vi "get_output_mode.vi"(8 "error in (no error)":errorcluster, 11 "connection ID":refnum<k5>) -> (0 "error out":errorcluster, 2 "Output mode":T1, 3 "connection ID out":refnum<k5>)   [LabVIEW 2018]
uses:
  typedefs/output_mode.ctl
panel:
  in  "Ouptut modes":string(combo)="0"
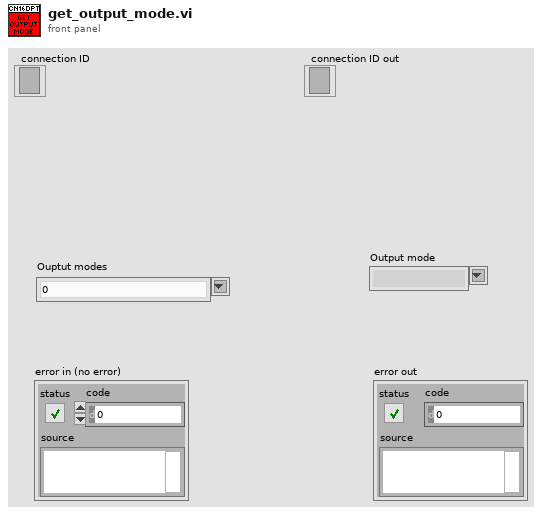
[diagram p1: front panel]
types:
  T1 = typedef "output_mode.ctl" = string
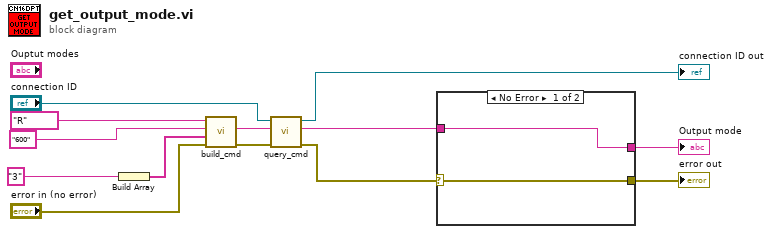
[diagram p0: block diagram]
diagram:
  n1 = Build Array("3" ("Output number")) -> (w2:string[])
  n2 = call "build_cmd.vi"("error in (no error)"="error in (no error)", "Parameter list"=w2, "Command ID"="600", "Command class"="R") -> ("error out"=w9:errorcluster, "Command"=w8:string)  [unwired: 6 in]
  n3 = call "query_cmd.vi"("error in (no error)"=w9, "Command"=w8, "connection ID"="connection ID") -> ("error out"=w7:errorcluster, "Response"=w6:string, "connection ID out"=→"connection ID out":refnum<k5>)  [unwired: 6 in]
  n4 = case shown="No Error" w7 {
    selector: w7 -> [w15 w16]
    tunnel: w6 -> [w14 _]
    tunnel: [w14 _] -> w4
    tunnel: [w15 w16] -> w5
    frame No Error {
    }
    frame Error {
    }
  }
  "error out" <- w5
  "Output mode" <- w4
